vi "GlobalMFC.vi"() -> ()   [LabVIEW 2013]
panel:
  in  "Array":dbl[](array[numeric])
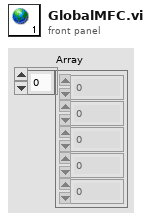
[diagram p1: front panel]
diagram:
